vi "Convert Ticks to Time.vi"(0 "Ticks":u64, 1 "Ticks 2":u64, 2 "Ticks 3":u64, 3 "Ticks 4":u64, 4 "Ticks 5":u64, 5 "Ticks 6":u64, 6 "Ticks 7":u64, 7 "Ticks 8":u64) -> (20 "Time":dbl[unit], 21 "Time  2":dbl[unit], 22 "Time  3":dbl[unit], 23 "Time  4":dbl[unit], 24 "Time  5":dbl[unit], 25 "Time  6":dbl[unit], 26 "Time  7":dbl[unit], 27 "Time  8":dbl[unit])   [LabVIEW 2009]
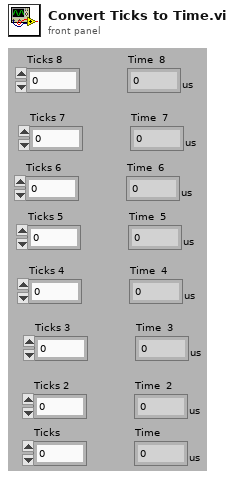
[diagram p1: front panel]
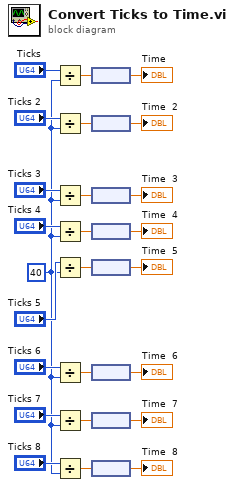
[diagram p0: block diagram]
diagram:
  w8 = u32 40 ("y")
  n1 = Divide(x="Ticks", y=w8) -> (x/y=w21:dbl)
  n2 = Divide(x="Ticks 2", y=w8) -> (x/y=w1:dbl)
  n3 = Divide(x="Ticks 3", y=w8) -> (x/y=w2:dbl)
  n4 = Divide(x="Ticks 4", y=w8) -> (x/y=w3:dbl)
  n5 = Divide(x="Ticks 5", y=w8) -> (x/y=w4:dbl)
  n6 = Divide(x="Ticks 6", y=w8) -> (x/y=w5:dbl)
  n7 = Divide(x="Ticks 7", y=w8) -> (x/y=w6:dbl)
  n8 = Divide(x="Ticks 8", y=w8) -> (x/y=w7:dbl)
  n9 = node(w21) -> (→"Time":dbl[unit])
  n10 = node(w1) -> (→"Time  2":dbl[unit])
  n11 = node(w2) -> (→"Time  3":dbl[unit])
  n12 = node(w3) -> (→"Time  4":dbl[unit])
  n13 = node(w4) -> (→"Time  5":dbl[unit])
  n14 = node(w5) -> (→"Time  6":dbl[unit])
  n15 = node(w6) -> (→"Time  7":dbl[unit])
  n16 = node(w7) -> (→"Time  8":dbl[unit])
